vi "Analytical Jacobian Matrix.vi"(0 "Euler angle":sgl[](array[numeric])) -> (1 "J":dbl[][](array[numeric]), 2 "J-":dbl[][](array[numeric]), 3 "JT":dbl[][](array[numeric]), 4 "J-T":dbl[][](array[numeric]))   [LabVIEW 2018]
uses:
  <vilib>/Analysis/baseanly.llb/Real Inverse Matrix.vi
  <vilib>/Analysis/Matrix/Numeric/Conversions/Matrix To Array - RM.vi
  <vilib>/Analysis/NI_AALBase.lvlib
  <vilib>/Analysis/Matrix/NI_Matrix.lvlib
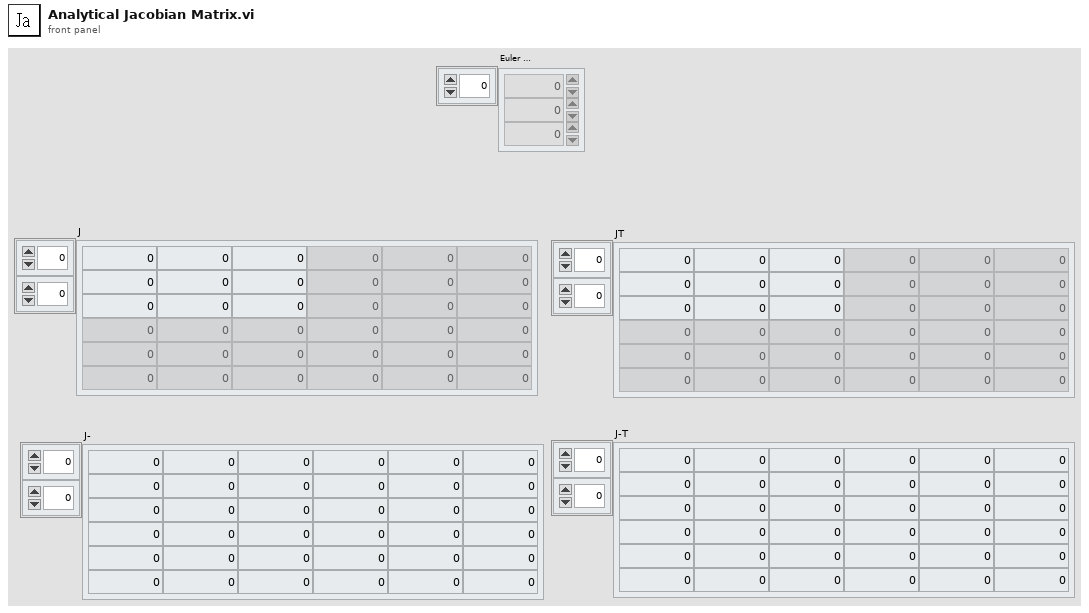
[diagram p1: front panel]
types:
  T1 = typedef "NI_Matrix.lvlib/RealMatrix.ctl" = dbl[][]
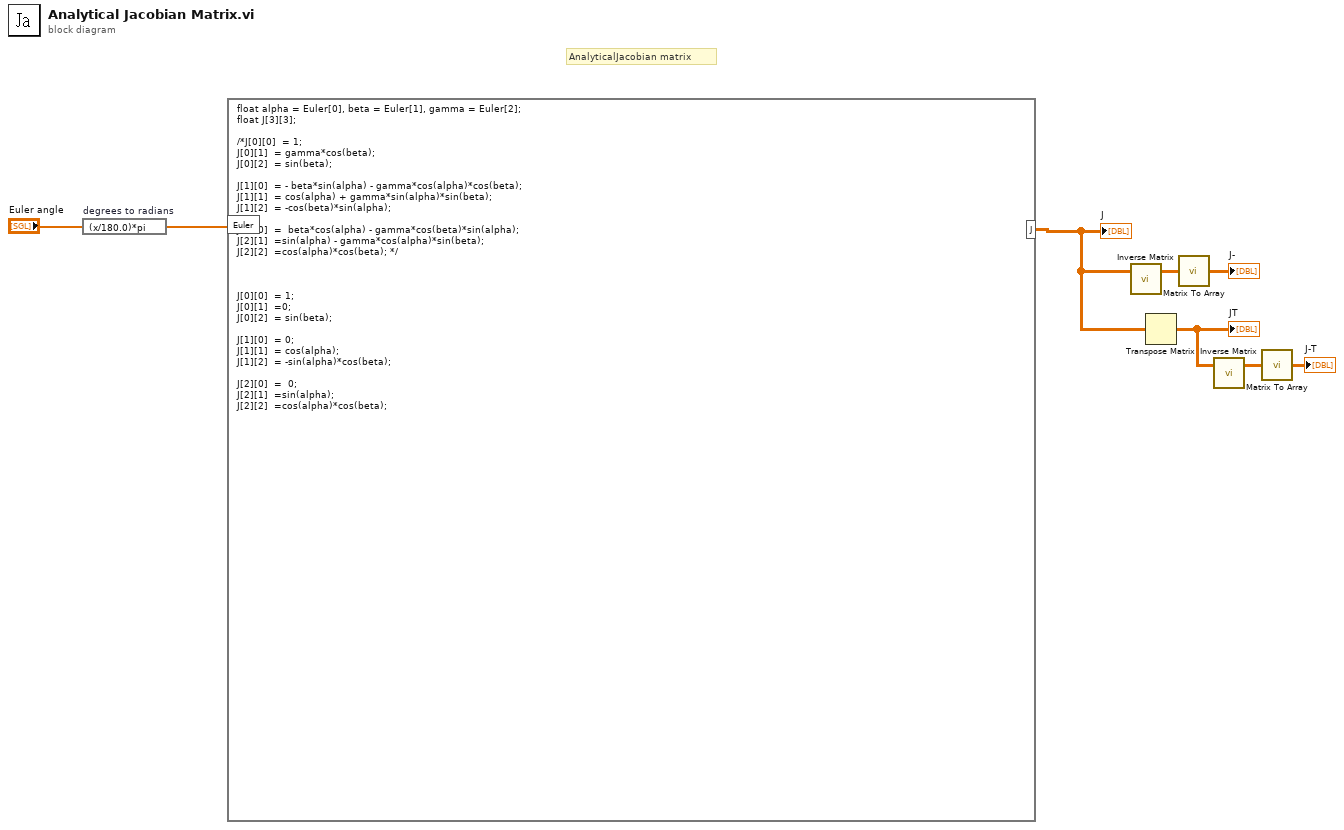
[diagram p0: block diagram]
diagram:
  # "AnalyticalJacobian matrix"
  n1 = expression code="(x/180.0)*pi" "degrees to radians"("Euler angle") -> (w2:sgl[])
  n2 = formula code="float alpha = Euler[0], beta = Euler[1], gamma = Euler[2];\nfloat J[3][3];\n\n/*J[0][0]  = 1;\nJ[0][1]  = gamma*cos(beta);\nJ[0][2]  = sin(beta);\n\nJ[1][0]  = - beta*sin(alpha) - gamma*cos(alpha)*cos(beta);\nJ[1][1]  = cos(alpha) + gamma*sin(alpha)*sin(beta);\nJ[1][2]  = -cos(beta)*sin(alpha);\n\nJ[2][0]  =  beta*cos(alpha) - gamma*cos(beta)*sin(alpha);\nJ[2][1]  =sin(alpha) - gamma*cos(alpha)*sin(beta);\nJ[2][2]  =cos(alpha)*cos(beta); */\n\n\n\nJ[0][0]  = 1;\nJ[0][1]  =0;\nJ[0][2]  = sin(beta);\n\nJ[1][0]  = 0;\nJ[1][1]  = cos(alpha);\nJ[1][2]  = -sin(alpha)*cos(beta);\n\nJ[2][0]  =  0;\nJ[2][1]  =sin(alpha);\nJ[2][2]  =cos(alpha)*cos(beta);"("Euler"=w2) -> ("J"=w4:dbl[][])
  "J" <- w4
  n3 = call-poly <vilib>:"Inverse Matrix.vi"("Input Matrix"=w4) -> ("Inverse Matrix"=w5:T1)  [unwired: 1 in, 1 out]
  n4 = Transpose Matrix(1:w4) -> (0:w8:dbl[][])
  "JT" <- w8
  n5 = call-poly <vilib>:"Matrix To Array.vi"("Real Matrix"=w5) -> ("Real 2D Array"=→"J-":dbl[][])
  n6 = call-poly <vilib>:"Inverse Matrix.vi"("Input Matrix"=w8) -> ("Inverse Matrix"=w7:T1)  [unwired: 1 in, 1 out]
  n7 = call-poly <vilib>:"Matrix To Array.vi"("Real Matrix"=w7) -> ("Real 2D Array"=→"J-T":dbl[][])
